vi "Initialize.vi"(7 "Channel Name":string="ActualValue.ch%d.AV", 8 "error in":errorcluster, 9 "Number of Channels":u32=1, 10 "Instance Name":string, 11 "Power Nominal Value in":refnum<class "Power Nominal Value.lvclass">) -> (0 "error out":errorcluster, 3 "Power Nominal Value out":refnum<class "Power Nominal Value.lvclass">)   [LabVIEW 2023, in "Power Nominal Value.lvclass"]
uses:
  Power Nominal Value.lvclass
  Parents/Nominal Value/Nominal Value.lvclass
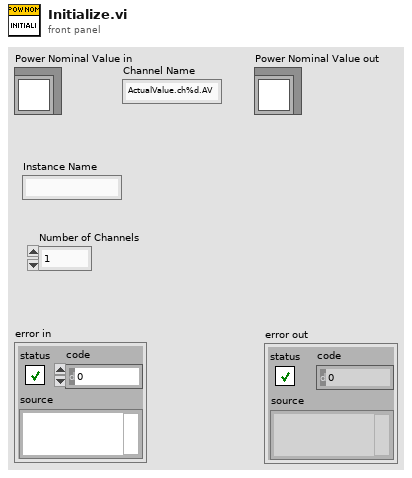
[diagram p1: front panel]
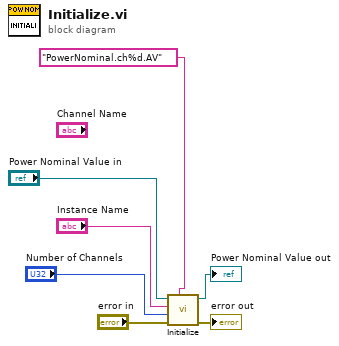
[diagram p0: block diagram]
diagram:
  n1 = call-parent "Initialize.vi"("Channel Name"="PowerNominal.ch%d.AV" ("ChannelName"), "error in"="error in", "Number of Channels"="Number of Channels", "Instance Name"="Instance Name", "Nominal Value in"="Power Nominal Value in") -> ("error out"=→"error out":errorcluster, "Nominal Value out"=→"Power Nominal Value out":refnum<class "Power Nominal Value.lvclass">)  [unwired: 5 in]
